vi "Carriage Intake Controller.vi"(8 "error in":errorcluster) -> ()   [LabVIEW 2018]
doc: "This VI executes continuously carrying out the current operation and responding to updates or new operations. It will often contain the timing or control code that is difficult to place directly in TeleOp. This VI generally opens all sensors and motors and isolates the rest of the robot code from knowing how the operations are carried out."
uses:
  <vilib>/Rock Robotics/WPI/Framework/Completion Status.ctl
  Carriage Intake Setpoints.ctl
  Carriage Intake Operations.ctl
  <vilib>/Rock Robotics/WPI/Solenoid/WPI_SolenoidChannel.ctl
  <vilib>/Rock Robotics/SystemInterfaces/DIO/FPGA_DIOChannel.ctl
  <vilib>/Rock Robotics/WPI/ThirdParty/Phoenix-LabVIEW/Motor Controller/Controls/CTRE_Phoenix_MotorControl_NeutralMode.ctl
  <vilib>/Rock Robotics/WPI/Solenoid/WPI_SolenoidValue.ctl
  <vilib>/Rock Robotics/WPI/Solenoid/WPI_SolenoidOpenDouble.vi
  <vilib>/Rock Robotics/WPI/Switch/WPI_SwitchOpenLimit.vi
  Framework/Robot Global Data.vi
  <vilib>/Rock Robotics/Network Tables/NT Write Boolean.vi
  <vilib>/Rock Robotics/WPI/Solenoid/WPI_SolenoidSetEnum.vi
panel:
  in  "Interactive Values":T1
  out "Current\nCmd":string
  in  "Buttons":cluster{"Execute Cmd":bool, "Abort Cmd":bool}
  out "Command Timing":cluster{"Start Time (ms)":u32, "Iterations":i32}
  out "Status":T3
  # "Tip: It may be helpful to observe inputs and sensor values.\nYou may also want to display tuning or debugging controls."
  # "Interactive Command: You may fill in the settings for a command\nand schedule it with the Execute button. You can observe and abort\nany command while fine tuning the code for the controller."
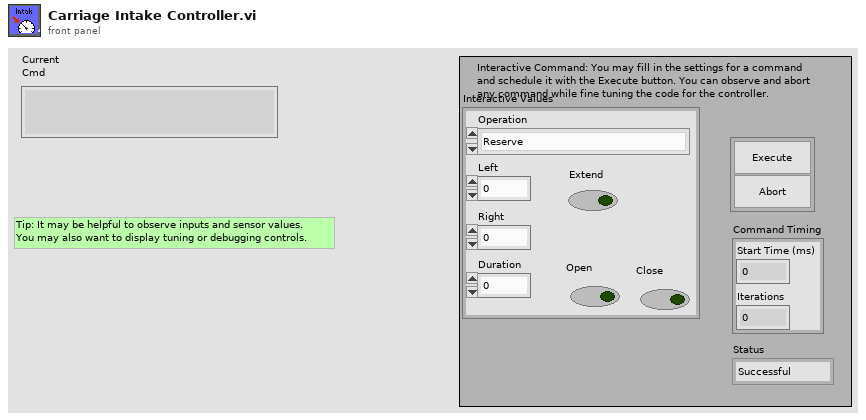
[diagram p1: front panel]
types:
  T1 = typedef "Carriage Intake Setpoints.ctl" = cluster{"Operation":T2, "Left":dbl, "Duration":dbl, "Extend":bool, "Open":bool, "Close":bool, "Right":dbl}
  T2 = typedef "Carriage Intake Operations.ctl" = enum16{"Reserve", "Read Current", "Immediate"}
  T3 = typedef "Completion Status.ctl" = enum16{"Successful", "Aborted", "Incomplete"}
  T4 = typedef "CTRE_Phoenix_MotorControl_NeutralMode.ctl" = enum8{"EEPROMSetting", "Override to Coast", "Override to Brake"}
  T5 = typedef "FPGA_DIOChannel.ctl" = enum8{"DIO 0", "DIO 1", "DIO 2", "DIO 3", "DIO 4", "DIO 5", "DIO 6", "DIO 7", "DIO 8", "DIO 9", "DIO MXP 0", "DIO MXP 1", "DIO MXP 2", "DIO MXP 3", "DIO MXP 4", "DIO MXP 5", "DIO MXP 6", "DIO MXP 7", "DIO MXP 8", "DIO MXP 9", "DIO MXP 10", "DIO MXP 11", "DIO MXP 12", "DIO MXP 13", "DIO MXP 14", "DIO MXP 15", "SPI Port CS1", "SPI Port CS2", "SPI Port CS3", "SPI Port MISO", "SPI Port MOSI", "Invalid"}
  T6 = typedef "WPI_SolenoidChannel.ctl" = enum8{"Solenoid 0", "Solenoid 1", "Solenoid 2", "Solenoid 3", "Solenoid 4", "Solenoid 5", "Solenoid 6", "Solenoid 7", "Invalid"}
  T7 = typedef "WPI_MotorControlDeviceRef.ctl" = cluster{"DeviceStatus":errorcluster, "Type":T8, "PWM":cluster{"PWM Channel":T9, "DeadBand":T10}, "CAN":cluster{"Device Number":u8, "SetOutput VI Ref":variant, "GetOutput VI Ref":variant, "Enable VI Ref":variant, "Disable VI Ref":variant, "Data":variant}, "Invert":bool, "DIO PWM":cluster{"PWM \"Enable\" Channel":T9, "DIOChannel":T5, "PWM Rate":dbl}}
  T8 = typedef "WPI_MotorControlType.ctl" = enum16{"PWM", "CAN", "DIO PWM"}
  T9 = typedef "FPGA_DIOPWMChannel.ctl" = enum8{"PWM 0", "PWM 1", "PWM 2", "PWM 3", "PWM 4", "PWM 5", "PWM 6", "PWM 7", "PWM 8", "PWM 9", "PWM MXP 0", "PWM MXP 1", "PWM MXP 2", "PWM MXP 3", "PWM MXP 4", "PWM MXP 5", "PWM MXP 6", "PWM MXP 7", "PWM MXP 8", "PWM MXP 9", "Invalid"}
  T10 = typedef "WPI_PWMDeadband.ctl" = cluster{"Name":string, "maxPositivePwm":i32, "minPositivePwm":i32, "centerPwm":i32, "maxNegativePwm":i32, "minNegativePwm":i32, "angularRange":u16}
  T11 = typedef "WPI_SolenoidDevRef.ctl" = cluster{"DevStatus":errorcluster, "Pneumatics Control Module":u8, "Forward Solenoid Channel":T6, "Reverse Solenoid Channel":T6}
  T12 = typedef "WPI_SwitchDevRef.ctl" = cluster{"DevStatus":errorcluster, "DIO Channel":T5, "CntIndex":T13, "Normally Closed":bool}
  T13 = typedef "FPGA_CounterCtrSystemIndex.ctl" = enum8{"Ctr 0", "Ctr 1", "Ctr 2", "Ctr 3", "Ctr 4", "Ctr 5", "Ctr 6", "Ctr 7", "Invalid"}
  T14 = typedef "Command Status Info.ctl" = cluster{"Name":string, "Status":T3, "notifier out":T15}
  T15 = typedef "Completion Notifier.ctl" = refnum<notifier>
  T16 = cluster{"Current Command":T1, "Command Timing":cluster{"Start Time (ms)":u32, "Iterations":i32}, "Command Arguments":cluster{"Command Info":T14, "Description":string, "Default Command":T1, "queue out":refnum<queue>, "Subsystem Name":string}}
  T17 = typedef "WPI_SolenoidValue.ctl" = enum16{"Off", "On", "Forward", "Reverse"}
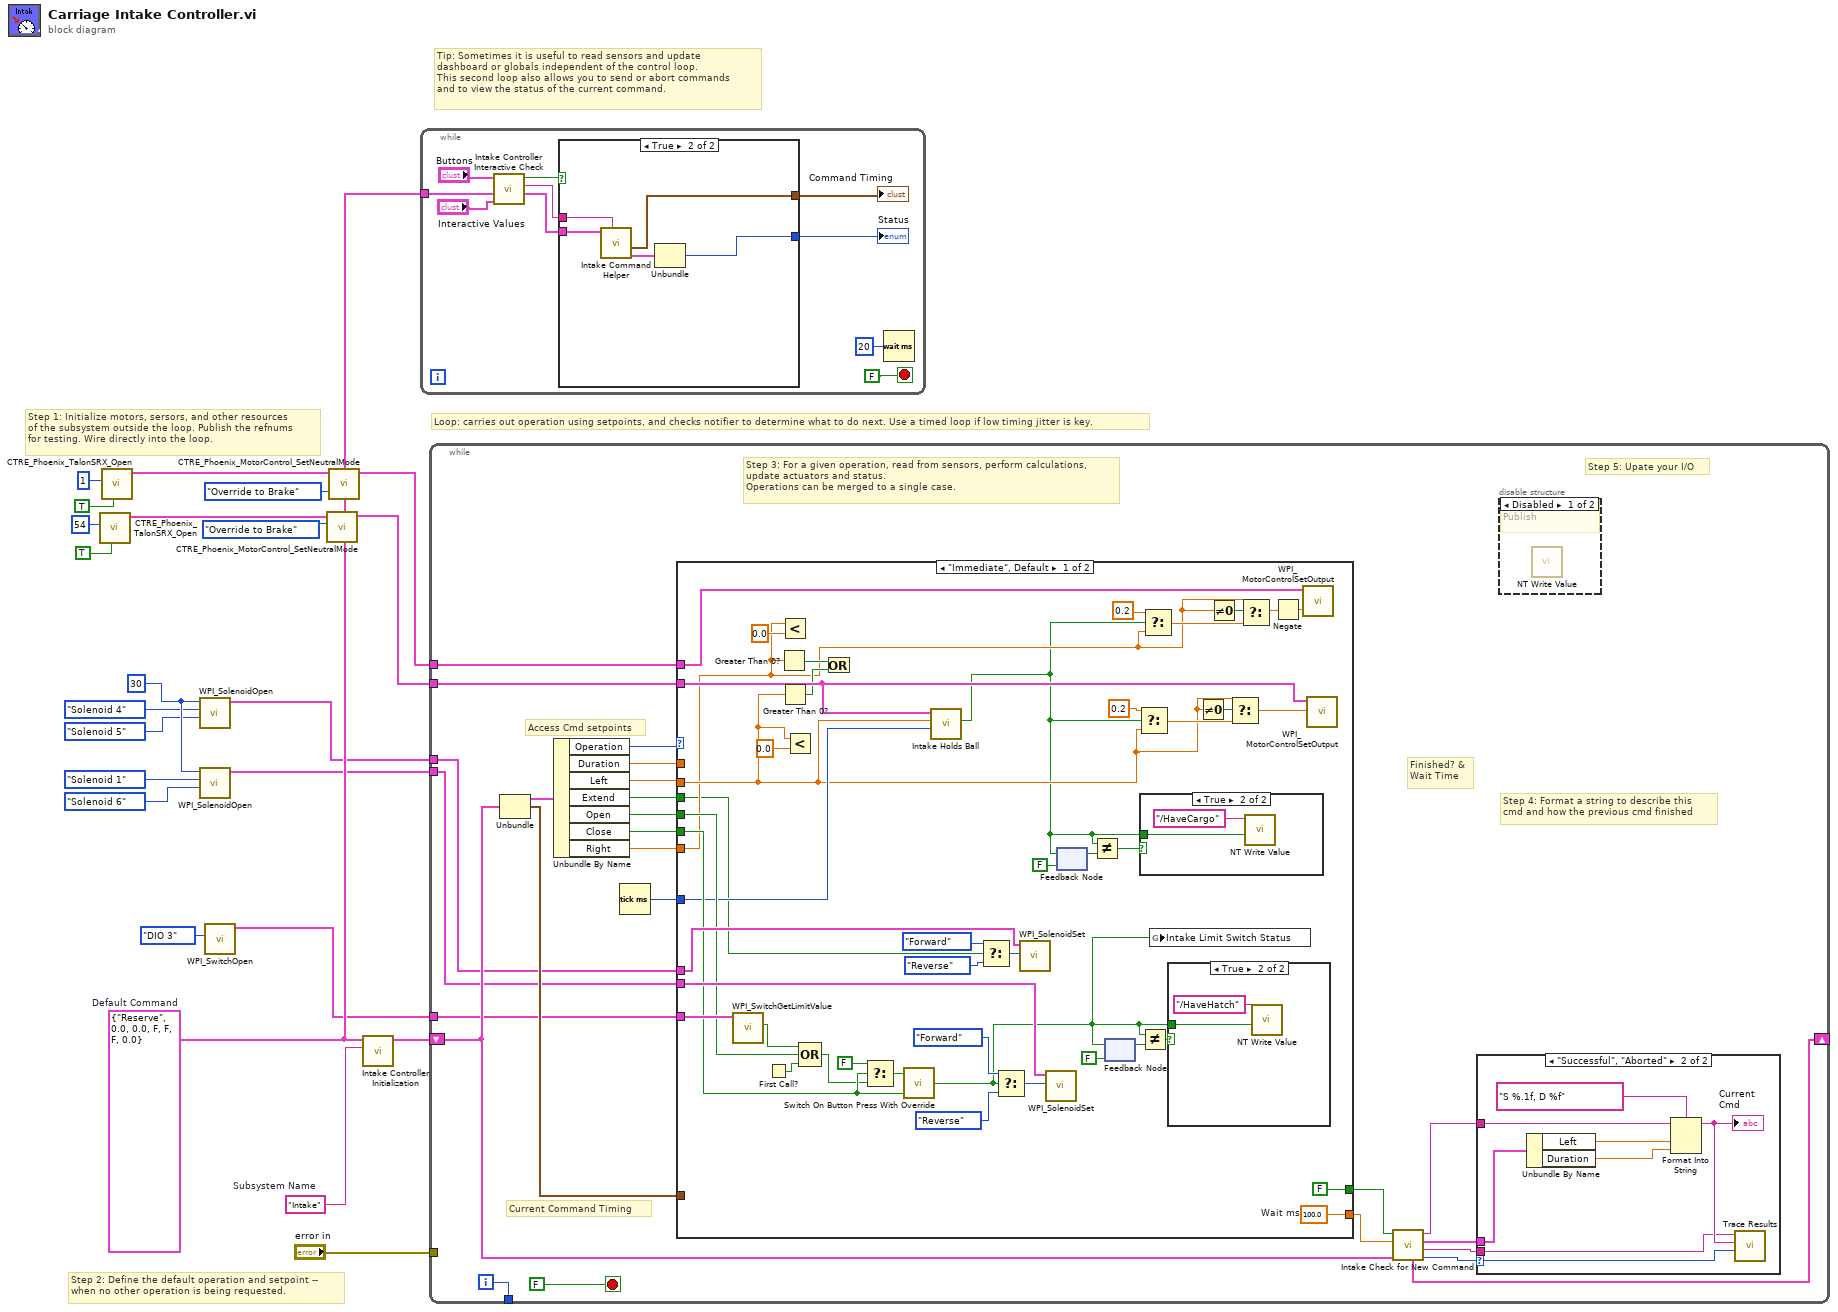
[diagram p0: block diagram]
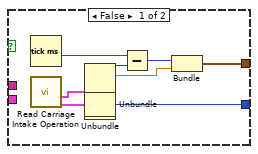
[diagram p2: hidden frame]
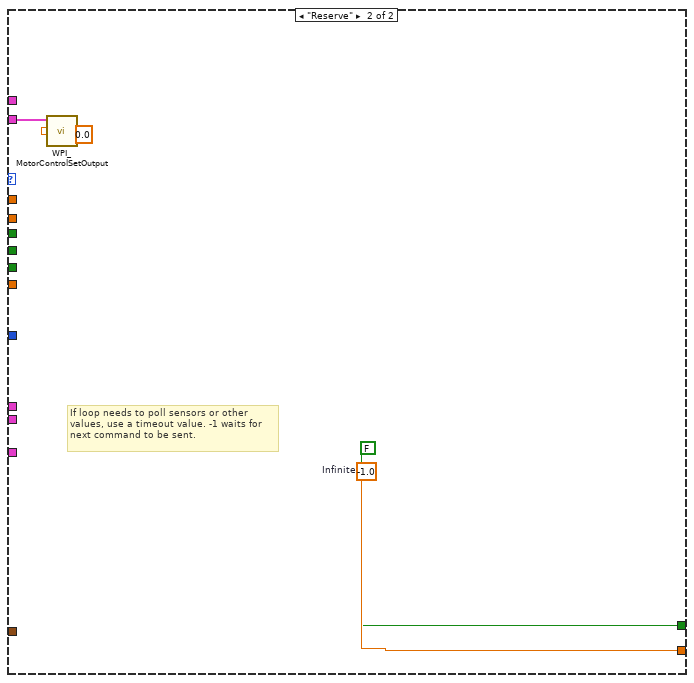
[diagram p5: hidden frame]
diagram:
  w15 = u8 30 ("Pneumatics Control Module (0)")
  w20 = T1 {"Operation"=enum."Reserve", "Left"=0.0, "Duration"=0.0, "Extend"=FALSE, "Open"=FALSE, "Close"=FALSE, "Right"=0.0}  # Default Command
  w21 = "Intake"  # Subsystem Name
  # "Tip: Sometimes it is useful to read sensors and update\ndashboard or globals independent of the control loop.\nThis second loop also allows you to send or abort commands\nand to view the status of the current command."
  # "Step 2: Define the default operation and setpoint --\nwhen no other operation is being requested."
  # "Step 1: Initialize motors, sersors, and other resources\nof the subsystem outside the loop. Publish the refnums\nfor testing. Wire directly into the loop."
  # "Loop: carries out operation using setpoints, and checks notifier to determine what to do next. Use a timed loop if low timing jitter is key."
  n1 = call <vilib>:"CTRE_Phoenix_TalonSRX_Open.vi"("Invert"=TRUE, "Device Number"=u8 54) -> ("CAN Talon SRX Ref"=w3:T7)  [unwired: 8 in, 1 out]
  n2 = call <vilib>:"CTRE_Phoenix_TalonSRX_Open.vi"("Invert"=TRUE, "Device Number"=u8 1) -> ("CAN Talon SRX Ref"=w6:T7)  [unwired: 8 in, 1 out]
  n3 = call-poly <vilib>:"WPI_SolenoidOpen.vi"("Reverse Solenoid Channel"=WPI_SolenoidChannel."Solenoid 5", "Forward Solenoid Channel"=WPI_SolenoidChannel."Solenoid 4", "Pneumatics Control Module (0)"=w15) -> ("SolenoidDevRef"=w17:T11)  [unwired: 7 in, 1 out]
  n4 = call-poly <vilib>:"WPI_SolenoidOpen.vi"("Reverse Solenoid Channel"=WPI_SolenoidChannel."Solenoid 6", "Forward Solenoid Channel"=WPI_SolenoidChannel."Solenoid 1", "Pneumatics Control Module (0)"=w15) -> ("SolenoidDevRef"=w16:T11)  [unwired: 7 in, 1 out]
  n5 = call-poly <vilib>:"WPI_SwitchOpen.vi"("DIO Channel"=FPGA_DIOChannel."DIO 3") -> ("SwitchDevRef"=w9:T12)  [unwired: 9 in, 1 out]
  n6 = call <vilib>:"CTRE_Phoenix_MotorControl_SetNeutralMode.vi"("Motor Control Neutral Mode"=CTRE_Phoenix_MotorControl_NeutralMode."Override to Brake", "PhoenixMotorControlDevRef"=w3) -> ("PhoenixMotorControlDevRef"=w1:T7)  [unwired: 8 in, 1 out]
  n7 = call <vilib>:"CTRE_Phoenix_MotorControl_SetNeutralMode.vi"("Motor Control Neutral Mode"=CTRE_Phoenix_MotorControl_NeutralMode."Override to Brake", "PhoenixMotorControlDevRef"=w6) -> ("PhoenixMotorControlDevRef"=w2:T7)  [unwired: 8 in, 1 out]
  n8 = call "Intake Controller Initialization.vi"("Subsystem Name"=w21, "Default Command"=w20) -> ("Current Command"=w22:T16)  [unwired: 9 in]
  n9 = while {
    tunnel: w20 -> [w30]
    stop <- FALSE stop-if-true
    n10 = call "Intake Controller Interactive Check.vi"("Interactive Command in"="Interactive Values", "Default Command"=w30, "Buttons"="Buttons") -> ("Interactive Command out"=w27:T1, "Trace String"=w28:string, "Schedule"=w29:bool)  [unwired: 6 in]
    n11 = case shown="True" w29 {
      tunnel: [w41 w46] -> w26
      tunnel: w27 -> [_ w44]
      tunnel: [w37 w42] -> w25
      tunnel: w28 -> [_ w45]
      frame False {
        n12 = Tick Count (ms)() -> (millisecond timer value=w36:u32)
        n13 = call "Read Carriage Intake Operation.vi"() -> ("Command Info"=w34:T14, "SubSystem Data"=w35:T1)  [unwired: 9 in, 1 out]
        n14 = Unbundle(w35) -> ("Operation"=w40:T2, "Left"=w38:dbl)  [unwired: 5 out]
        n15 = Unbundle(w34) -> ("Status"=w41:T3)  [unwired: 2 out]
        n16 = Subtract(x=w36, y=w40) -> (x-y=w39:u32)
        n17 = Bundle(w39, "Left"=w38) -> (w37:cluster{u32, "Left":dbl})  [unwired: 1 in]
      }
      frame True {
        n18 = call "Intake Command Helper.vi"("Description"=w45, "SubSystem Data"=w44) -> ("Command Info Out"=w43:T14, "Command Timing"=w42:cluster{"Start Time (ms)":u32, "Iterations":i32})  [unwired: 7 in, 1 out]
        n19 = Unbundle(w43) -> ("Status"=w46:T3)  [unwired: 2 out]
      }
    }
    "Status" <- w26
    "Command Timing" <- w25
    n20 = Wait (ms)(milliseconds to wait=u32 20) -> ()  [unwired: 1 out]
  }
  n21 = while {
    shift-right: [w63] -> _
    shift-left: w22 -> [w56]
    tunnel: [w70] -> _
    tunnel: "error in" -> [_]
    tunnel: w1 -> [w55]
    tunnel: w17 -> [w53]
    tunnel: w16 -> [w52]
    tunnel: w9 -> [w51]
    tunnel: w2 -> [w47]
    i -> [w70]
    stop <- FALSE stop-if-true
    # "Step 5: Upate your I/O"
    # "Step 4: Format a string to describe this\ncmd and how the previous cmd finished"
    # "Current Command Timing"
    # "Access Cmd setpoints"
    # "Finished? &\nWait Time"
    # "Step 3: For a given operation, read from sensors, perform calculations,\nupdate actuators and status.\nOperations can be merged to a single case."
    n22 = Unbundle(w56) -> ("Current Command"=w69:T1, "Command Timing"=w65:cluster{"Start Time (ms)":u32, "Iterations":i32})  [unwired: 1 out]
    n23 = Unbundle By Name(w69) -> ("Operation"=w68:T2, "Duration"=w67:dbl, "Left"=w64:dbl, "Extend"=w54:bool, "Open"=w50:bool, "Close"=w49:bool, "Right"=w48:dbl)
    n24 = Tick Count (ms)() -> (millisecond timer value=w66:u32)
    n25 = case shown="\"Immediate\", Default" w68 {
      tunnel: [w116 w124] -> w61
      tunnel: [FALSE ("ignore previous (F)") FALSE ("ignore previous (F)")] -> w62
      tunnel: w65 -> [_ _]
      tunnel: w67 -> [_ _]
      tunnel: w66 -> [w84 _]
      tunnel: w64 -> [w80 _]
      tunnel: w55 -> [w105 w122]
      tunnel: w54 -> [w75 _]
      tunnel: w53 -> [w112 _]
      tunnel: w52 -> [w108 _]
      tunnel: w51 -> [w109 _]
      tunnel: w50 -> [w94 _]
      tunnel: w49 -> [w95 _]
      tunnel: w48 -> [w78 _]
      tunnel: w47 -> [w85 _]
      frame "Immediate", Default {
        w116 = 100.0  # Wait ms
        n26 = call <vilib>:"WPI_SwitchGetLimitValue.vi"("SwitchDevRef"=w109) -> ("Switch Pressed"=w76:bool)  [unwired: 8 in, 2 out]
        n27 = First Call?() -> (First Call?: T/F=w92:bool)
        n28 = Greater Than 0?(x=w78) -> (x > 0?=w83:bool)
        n29 = Less?(x=w78, y=0.0) -> ()  [unwired: 1 out]
        n30 = Greater Than 0?(x=w80) -> (x > 0?=w82:bool)
        n31 = Less?(x=w80, y=0.0) -> ()  [unwired: 1 out]
        n32 = Compound Arithmetic op=OR(w76, w94, w92) -> (w93:bool)
        n33 = Or(x=w83, y=w82) -> ()  [unwired: 1 out]
        n34 = Select(t=FALSE ("f"), s=w95, f=w93) -> (s? t:f=w97:bool)
        n35 = call "Switch On Button Press With Override.vi"("Override False"=w95, "Override True"=w97) -> ("Output"=w74:bool)  [unwired: 1 in]
        n36 = call "Intake Holds Ball.vi"("time"=w84, "motor power"=w80, "PhoenixMotorControlDevRef"=w105) -> ("has ball?"=w77:bool)  [unwired: 8 in]
        n37 = Select(t=WPI_SolenoidValue."Forward" ("Value"), s=w75, f=WPI_SolenoidValue."Reverse" ("Value")) -> (s? t:f=w115:T17)
        n38 = Select(t=WPI_SolenoidValue."Forward" ("Value"), s=w74, f=WPI_SolenoidValue."Reverse" ("Value")) -> (s? t:f=w110:T17)
        n39 = call-poly <vilib>:"WPI_SolenoidSet.vi"("Value"=w115, "SolenoidDevRef"=w112) -> ()  [unwired: 8 in, 2 out]
        n40 = call-poly <vilib>:"WPI_SolenoidSet.vi"("Value"=w110, "SolenoidDevRef"=w108) -> ()  [unwired: 8 in, 2 out]
        n41 = feedback-in #1(w77) -> ()
        n42 = feedback #1(FALSE ("has ball?")) -> (w102:bool)
        n43 = Not Equal?(x=w77, y=w102) -> (x != y?=w101:bool)
        n44 = feedback #2(FALSE ("has ball?")) -> (w100:bool)
        n45 = feedback-in #2(w74) -> ()
        n46 = Select(t=0.2, s=w77, f=w80) -> (s? t:f=w87:dbl)
        n47 = case shown="True" w101 {
          tunnel: w77 -> [_ w119]
          frame False {
          }
          frame True {
            n48 = call-poly <vilib>:"NT Write Value.vi"("Boolean"=w119, "Name"="/HaveCargo") -> ()  [unwired: 9 in, 1 out]
          }
        }
        n49 = Not Equal?(x=w74, y=w100) -> (x != y?=w98:bool)
        n50 = Select(t=0.2, s=w77, f=w78) -> (s? t:f=w89:dbl)
        n51 = global write "Robot Global Data.vi" "Intake Limit Switch Status"(w74) -> ()
        n52 = case shown="True" w98 {
          tunnel: w74 -> [_ w118]
          frame False {
          }
          frame True {
            n53 = call-poly <vilib>:"NT Write Value.vi"("Boolean"=w118, "Name"="/HaveHatch") -> ()  [unwired: 9 in, 1 out]
          }
        }
        n54 = Not Equal To 0?(x=w80) -> (x != 0?=w88:bool)
        n55 = Not Equal To 0?(x=w78) -> (x != 0?=w90:bool)
        n56 = Select(t=w80, s=w88, f=w87) -> (s? t:f=w86:dbl)
        n57 = Select(t=w78, s=w90, f=w89) -> (s? t:f=w73:dbl)
        n58 = Negate(x=w73) -> (-x=w72:dbl)
        n59 = call <vilib>:"WPI_MotorControlSetOutput.vi"("Output"=w72, "MotorControlDevRef"=w85) -> ()  [unwired: 7 in, 3 out]
        n60 = call <vilib>:"WPI_MotorControlSetOutput.vi"("Output"=w86, "MotorControlDevRef"=w105) -> ()  [unwired: 7 in, 3 out]
      }
      frame "Reserve" {
        w124 = -1.0  # Infinite
        # "If loop needs to poll sensors or other\nvalues, use a timeout value. -1 waits for\nnext command to be sent."
        n61 = call <vilib>:"WPI_MotorControlSetOutput.vi"("Output"=0.0, "MotorControlDevRef"=w122) -> ()  [unwired: 7 in, 3 out]
      }
    }
    n62 = call "Intake Check for New Command.vi"("Current Command"=w56, "Wait time (ms)"=w61, "Finished?"=w62) -> ("Completion"=w57:T3, "Subsystem Name"=w58:string, "Current Command"=w59:T1, "Initial Trace String"=w60:string, "NextCommand"=w63:T16)  [unwired: 4 in]
    n63 = case shown="\"Successful\", \"Aborted\"" w57 {
      selector: w57 -> [_ w132]
      tunnel: w60 -> [_ w128]
      tunnel: w59 -> [_ w129]
      tunnel: w58 -> [_ w125]
      frame "Incomplete", Default {
        # "Continuing current command"
      }
      frame "Successful", "Aborted" {
        # "Report and setup for next command"
        n64 = Unbundle By Name(w129) -> ("Left"=w131:dbl, "Duration"=w126:dbl)
        n65 = Format Into String(format string="S %.1f, D %f", initial string=w128, w131, w126) -> (resulting string=w127:string)  [unwired: 1 in, 1 out]
        "Current\nCmd" <- w127
        n66 = call <vilib>:"Trace Results.vi"("Status of previous command"=w132, "Description"=w127, "Subsystem"=w125) -> ()  [unwired: 9 in]
      }
    }
    n67 = disable-structure shown="Disabled" {
      frame Disabled {
        # "Publish"
        n68 = call-poly <vilib>:"NT Write Value.vi"() -> ()  [unwired: 11 in, 1 out]
      }
      frame Enabled {
      }
    }
  }
